vi "create test image for tracking.vi"(8 "error in (no error)":errorcluster, 11 "Image Src":T1) -> (0 "error out":errorcluster, 3 "Image Dst Out":T1)   [LabVIEW 2020]
uses:
  <vilib>/vision/Image Controls.llb/IMAQ Image.ctl
  <vilib>/vision/NI_Vision_Development_Module.lvlib
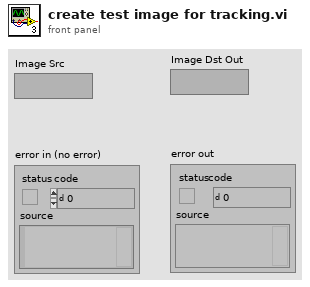
[diagram p1: front panel]
types:
  T1 = typedef "IMAQ Image.ctl" = refnum<image>
  T2 = typedef "Image Type" = u32
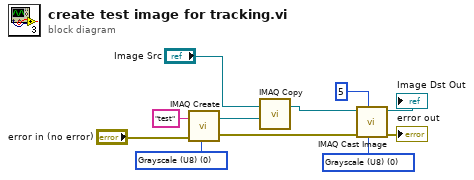
[diagram p0: block diagram]
diagram:
  w10 = T2 0 items=["Grayscale (U8)", "Grayscale (I16)", "Grayscale (SGL)", "Complex (CSG)", "RGB (U32)", "HSL (U32)", "RGB (U64)", "Grayscale (U16)"] ("Image Type")
  w11 = T2 0 items=["Grayscale (U8)", "Grayscale (I16)", "Grayscale (SGL)", "Complex (CSG)", "RGB (U32)", "HSL (U32)", "RGB (U64)", "Grayscale (U16)"] ("Image Type")
  n1 = call "IMAQ Create"("Image Name"="test", "Image Type"=w10, "error in (no error)"="error in (no error)") -> ("New Image"=w9:T1, "error out"=w6:errorcluster)  [unwired: 2 in]
  n2 = call "IMAQ Copy"("Image Dst"=w9, "Image Src"="Image Src") -> ("Image Dst Out"=w8:T1)  [unwired: 4 in, 1 out]
  n3 = call "IMAQ Cast Image"("Image Type"=w11, "# Shifts"=5, "error in (no error)"=w6, "Image Src"=w8) -> ("error out"=→"error out":errorcluster, "Image Dst Out"=→"Image Dst Out":T1)  [unwired: 6 in]
